vi "Find Enum Member Names.vi"(6 "Enum TypeName":string, 8 "error in":errorcluster, 11 "Doc Ref":refnum<k20>) -> (0 "error out":errorcluster, 2 "EnumMembers":string[](array[string]))   [LabVIEW 2026, in "Plugin XML Parser.lvlib"]
uses:
  Plugin XML Parser.lvlib
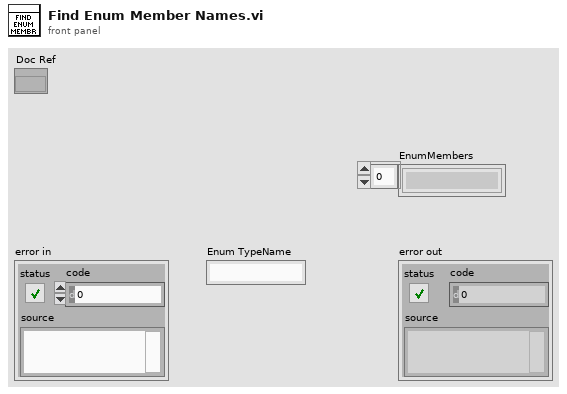
[diagram p1: front panel]
types:
  T1 = cluster{"TypeName":string, "EnumMembers":string[]}[]
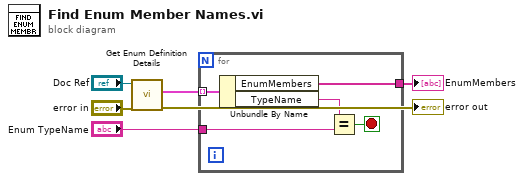
[diagram p0: block diagram]
diagram:
  n1 = call "Get Enum Definition Details.vi"("error in"="error in", "Doc Ref"="Doc Ref") -> ("error out"=→"error out":errorcluster, "Enum Definition Details"=w4:T1)  [unwired: 8 in]
  n2 = for {
    tunnel: w4 -> [w11] mode=indexing
    tunnel: "Enum TypeName" -> [w9]
    tunnel: [w7] -> w2
    stop <- w8 stop-if-true
    n3 = Unbundle By Name(w11) -> ("EnumMembers"=w7:string[], "TypeName"=w10:string)
    n4 = Equal?(x=w10, y=w9) -> (x = y?=w8:bool)
  }
  "EnumMembers" <- w2
